vi "Get State.vi"(8 "error in (no error)":errorcluster, 11 "Spectrum Recorder in":refnum<class "Spectrum Recorder too.lvclass">) -> (0 "error out":errorcluster, 1 "Result ready":bool, 2 "Armed":bool, 3 "Spectrum Recorder out":refnum<class "Spectrum Recorder too.lvclass">)   [LabVIEW 2016, in "Spectrum Recorder too.lvclass"]
uses:
  Spectrum Recorder too.lvclass
  C:/github/Measure_core/Worker/Worker.lvclass
  C:/github/Measure_core/Instrument Actor/Instrument Actor.lvclass
  Measure_core/Worker/Worker.lvclass/Worker.ctl
  Spectrum Recorder too.lvclass/Spectrum Recorder too.ctl
  Measure_core/Template Module/Read Active.vi
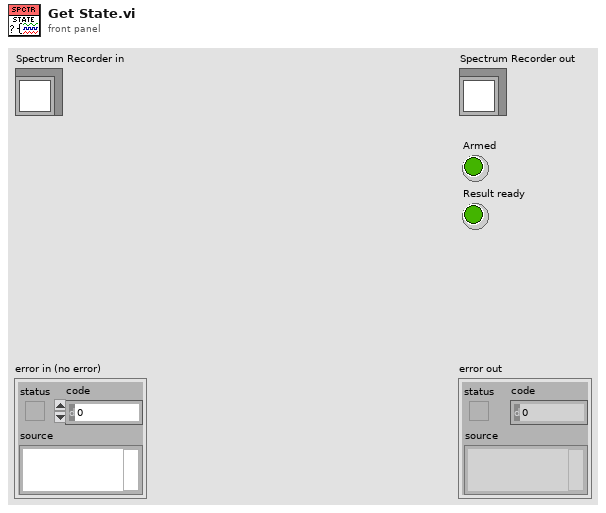
[diagram p1: front panel]
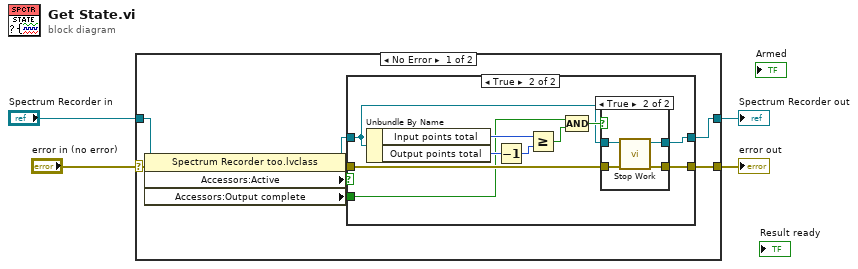
[diagram p0: block diagram]
diagram:
  n1 = case shown="No Error" "error in (no error)" {
    selector: "error in (no error)" -> [w11 w32]
    tunnel: [w10 w32] -> w3
    tunnel: [w12 w31] -> w1
    tunnel: "Spectrum Recorder in" -> [w8 w31]
    frame No Error {
      n2 = property class="Spectrum Recorder too.lvclass"(reference=w8, error in=w11) -> (reference out=w7:refnum<class "Spectrum Recorder too.lvclass">, error out=w9:errorcluster, "Accessors:Active"=w6:bool, "Accessors:Output complete"=w5:bool)
      n3 = case shown="True" w6 {
        tunnel: w7 -> [w13 w20]
        tunnel: w9 -> [w14 w19]
        tunnel: [w14 w18] -> w10
        tunnel: [w13 w17] -> w12
        tunnel: w5 -> [_ w15]
        frame False {
        }
        frame True {
          n4 = Unbundle By Name(w20) -> ("Input points total"=w23:i64, "Output points total"=w22:i64)
          n5 = Decrement(x=w22) -> (x-1=w16:i64)
          n6 = Greater Or Equal?(x=w23, y=w16) -> (x >= y?=w21:bool)
          n7 = Compound Arithmetic op=AND(w15, w21) -> (w24:bool)
          n8 = case shown="True" w24 {
            tunnel: w20 -> [w26 w30]
            tunnel: w19 -> [w25 w29]
            tunnel: [w25 w28] -> w18
            tunnel: [w26 w27] -> w17
            frame False {
            }
            frame True {
              n9 = call-dynamic "Stop Work.vi"("error in (no error)"=w29, "Spectrum Recorder in"=w30) -> ("error out"=w28:errorcluster, "Spectrum Recorder out"=w27:refnum<class "Spectrum Recorder too.lvclass">)  [unwired: 8 in]
            }
          }
        }
      }
    }
    frame Error {
    }
  }
  "error out" <- w3
  "Spectrum Recorder out" <- w1
